vi "Get Coverage Percentage.vi"(8 "error in (no error)":errorcluster, 10 "VI Path":path, 11 "Fake Code Coverage in":refnum<class "Fake Code Coverage.lvclass">) -> (0 "error out":errorcluster, 2 "Coverage Percentage":dbl, 3 "Fake Code Coverage out":refnum<class "Fake Code Coverage.lvclass">)   [LabVIEW 2017, in "Cobertura.Tests.lvlib" / "Fake Code Coverage.lvclass"]
doc: "Returns the code coverage percentage for a given VI."
uses:
  Fake Code Coverage.lvclass
  Fake Code Coverage.lvclass/Fake Code Coverage.ctl
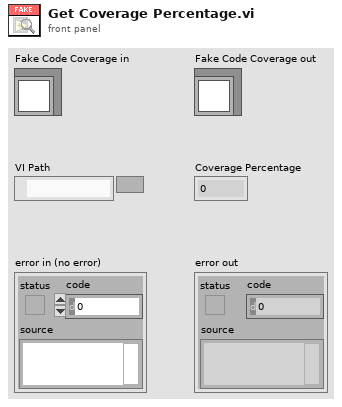
[diagram p1: front panel]
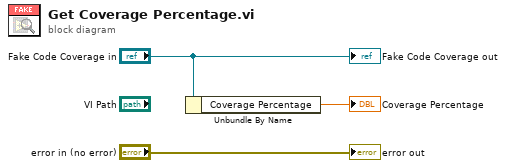
[diagram p0: block diagram]
diagram:
  n1 = Unbundle By Name("Fake Code Coverage in") -> ("Coverage Percentage"=→"Coverage Percentage":dbl)
  "error out" <- "error in (no error)"
  "Fake Code Coverage out" <- "Fake Code Coverage in"
